vi "Laser line to resource name.vi"(8 "error in (no error)":errorcluster, 10 "Laser line":T1 items=["405nm"=4, "445nm"=16, "491nm"=18, "515nm"=9, "561nm"=19], 11 "Cobolt in":refnum<class "Cobolt.lvclass">) -> (0 "error out":errorcluster, 2 "VISA resource":string, 3 "Cobolt out":refnum<class "Cobolt.lvclass">)   [LabVIEW 2012, in "Cobolt.lvclass"]
uses:
  Cobolt.lvclass
  laser lines.ctl
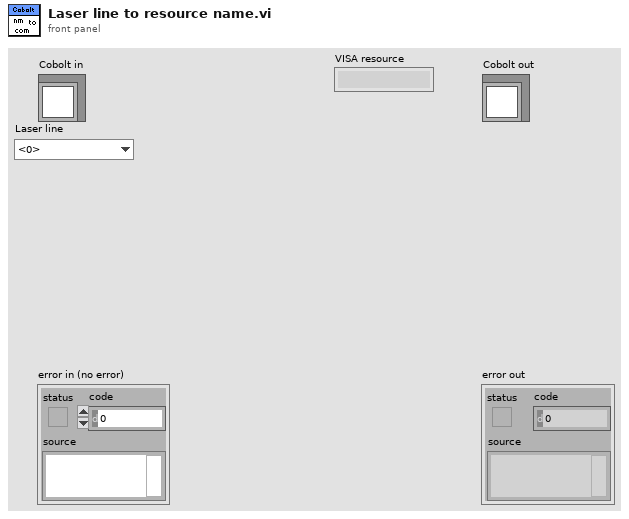
[diagram p1: front panel]
types:
  T1 = typedef "Cobolt.lvclass/laser lines.ctl" = u16
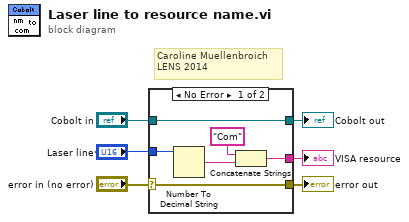
[diagram p0: block diagram]
diagram:
  # "Caroline Muellenbroich\nLENS 2014"
  n1 = case shown="No Error" "error in (no error)" {
    selector: "error in (no error)" -> [w12 w14]
    tunnel: [w12 w14] -> w5
    tunnel: [w8 w13] -> w3
    tunnel: "Cobolt in" -> [w8 w13]
    tunnel: [w9 _] -> w2
    tunnel: "Laser line" -> [w7 _]
    frame No Error {
      n2 = Number To Decimal String(number=w7) -> (decimal integer string=w10:string)  [unwired: 1 in]
      n3 = Concatenate Strings("Com" ("string"), w10) -> (w9:string)
    }
    frame Error {
    }
  }
  "error out" <- w5
  "Cobolt out" <- w3
  "VISA resource" <- w2
